vi "for.vi"() -> ()   [LabVIEW 2020]
panel:
  out "Array":i32[](array[numeric])
  out "Thermometer":dbl(slide) scale=0.0..100.0
  out "x+1":i32
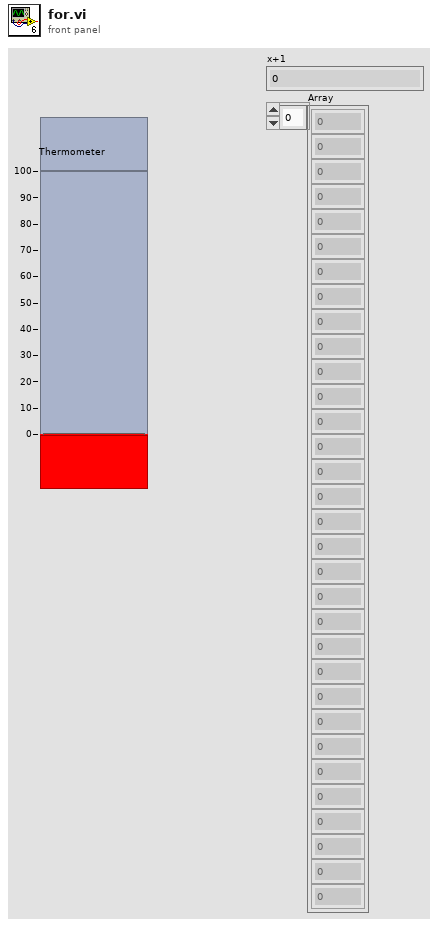
[diagram p1: front panel]
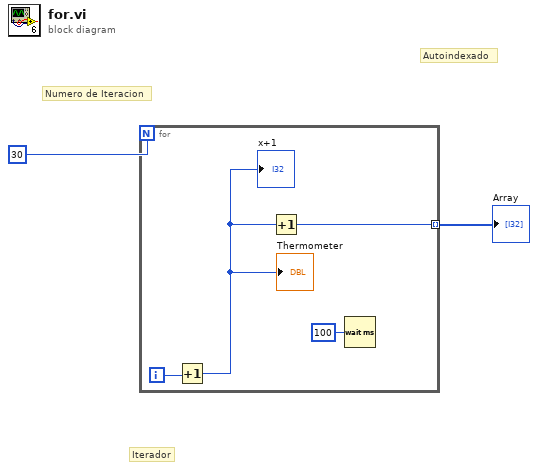
[diagram p0: block diagram]
diagram:
  # "Autoindexado"
  # "Numero de Iteracion"
  # "Iterador"
  n1 = for {
    N: 30 -> [_]
    tunnel: [w3] -> w1 mode=indexing
    i -> [w6]
    n2 = Increment(x=w6) -> (x+1=w4:i32)
    "x+1" <- w4
    "Thermometer" <- w4
    n3 = Increment(x=w4) -> (x+1=w3:i32)
    n4 = Wait (ms)(milliseconds to wait=u32 100) -> ()  [unwired: 1 out]
  }
  "Array" <- w1
